vi "Dec_to_ASCII_char.vi"(11 "SetPoint":ext) -> (3 "字符串":string)   [LabVIEW 2014]
panel:
  out "字符串 2":string
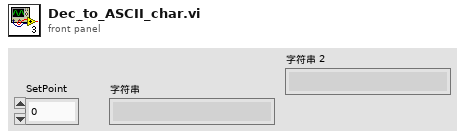
[diagram p1: front panel]
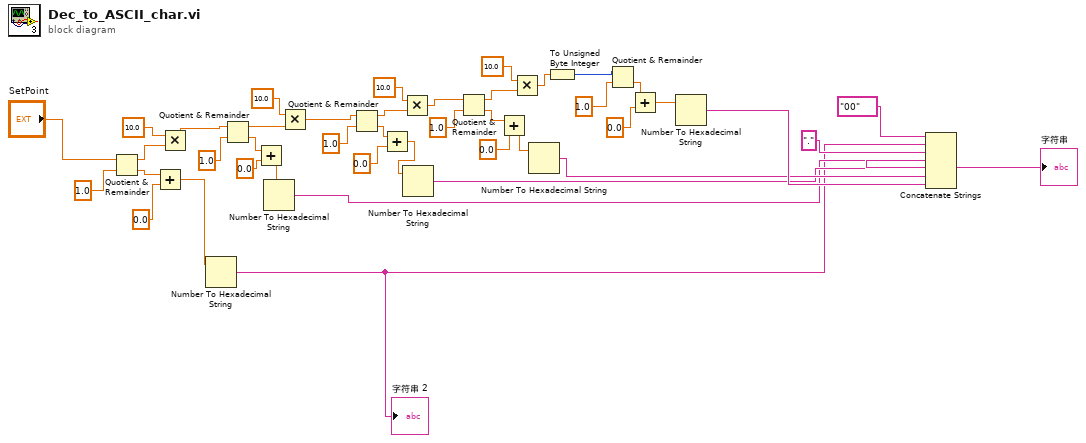
[diagram p0: block diagram]
diagram:
  n1 = Quotient & Remainder(x="SetPoint", y=1.0) -> (x-y*floor(x/y)=w7:ext, floor(x/y)=w4:ext)
  n2 = Add(x=w4, y=0.0) -> (x+y=w6:ext)
  n3 = Multiply(x=10.0, y=w7) -> (x*y=w9:ext)
  n4 = Number To Hexadecimal String(2:w6) -> (0:w1:string)  [unwired: 1 in]
  "字符串 2" <- w1
  n5 = Quotient & Remainder(x=w9, y=1.0) -> (x-y*floor(x/y)=w12:ext, floor(x/y)=w21:ext)
  n6 = Add(x=w21, y=0.0) -> (x+y=w23:ext)
  n7 = Number To Hexadecimal String(2:w23) -> (0:w33:string)  [unwired: 1 in]
  n8 = Multiply(x=10.0, y=w12) -> (x*y=w13:ext)
  n9 = Quotient & Remainder(x=w13, y=1.0) -> (x-y*floor(x/y)=w15:ext, floor(x/y)=w24:ext)
  n10 = Add(x=w24, y=0.0) -> (x+y=w26:ext)
  n11 = Multiply(x=10.0, y=w15) -> (x*y=w17:ext)
  n12 = Number To Hexadecimal String(2:w26) -> (0:w34:string)  [unwired: 1 in]
  n13 = Quotient & Remainder(x=w17, y=1.0) -> (x-y*floor(x/y)=w19:ext, floor(x/y)=w27:ext)
  n14 = Add(x=w27, y=0.0) -> (x+y=w29:ext)
  n15 = Multiply(x=10.0, y=w19) -> (x*y=w38:ext)
  n16 = Number To Hexadecimal String(2:w29) -> (0:w35:string)  [unwired: 1 in]
  n17 = To Unsigned Byte Integer(number=w38) -> (unsigned 8bit integer=w40:u8)
  n18 = Quotient & Remainder(x=w40, y=1.0) -> (floor(x/y)=w39:dbl)  [unwired: 1 out]
  n19 = Add(x=w39, y=0.0) -> (x+y=w31:dbl)
  n20 = Number To Hexadecimal String(2:w31) -> (0:w36:string)  [unwired: 1 in]
  n21 = Concatenate Strings("00", w1, "." ("字符串"), w33, w34, w35, w36) -> (→"字符串":string)
